vi "HGCalSensorTestingPanel3.vi"() -> ()   [LabVIEW 2015]
uses:
  <vilib>/Utility/file.llb/Read Delimited Spreadsheet (DBL).vi
  <vilib>/Utility/file.llb/Write Delimited Spreadsheet (string).vi
panel:
  out "XY Graph 3":cluster{"Y":dbl[], "Y":dbl[]}[](graph)
  out "HP count":u32
  in  "HP read count":u32
  in  "HP VISA":refnum<visa-resource-name>
  out "K237 count":u32
  in  "K237 VISA":refnum<visa-resource-name>
  out "XY Graph 2":cluster{"Y":dbl[], "Y":dbl[]}[](graph)
  out "return count 5":u32
  in  "write buffer 2":string
  out "return count 4":u32
  in  "QT VISA":refnum<visa-resource-name>
  in  "write buffer":string
  out "return count 3":u32
  in  "byte count 2":u32
  out "XY Graph":cluster{"Y":dbl[], "Y":dbl[]}[](graph)
  out "return count":u32
  in  "K706 VISA":refnum<visa-resource-name>
  in  "Measurement Data":string[][](table)
  in  "OK Button":bool
  in  "Delay (s):":dbl
  in  "Channel:":dbl
  in  "Voltage (V):":dbl
  out "Channel:":dbl format="%#3_6g"
  out "mV(nA)":dbl
  out "pF":dbl
  out "V":dbl
  out "nA":dbl
  # "C"
  # "A"
  # "V"
  # "1M"
  # "1M"
  # "Single Measurement"
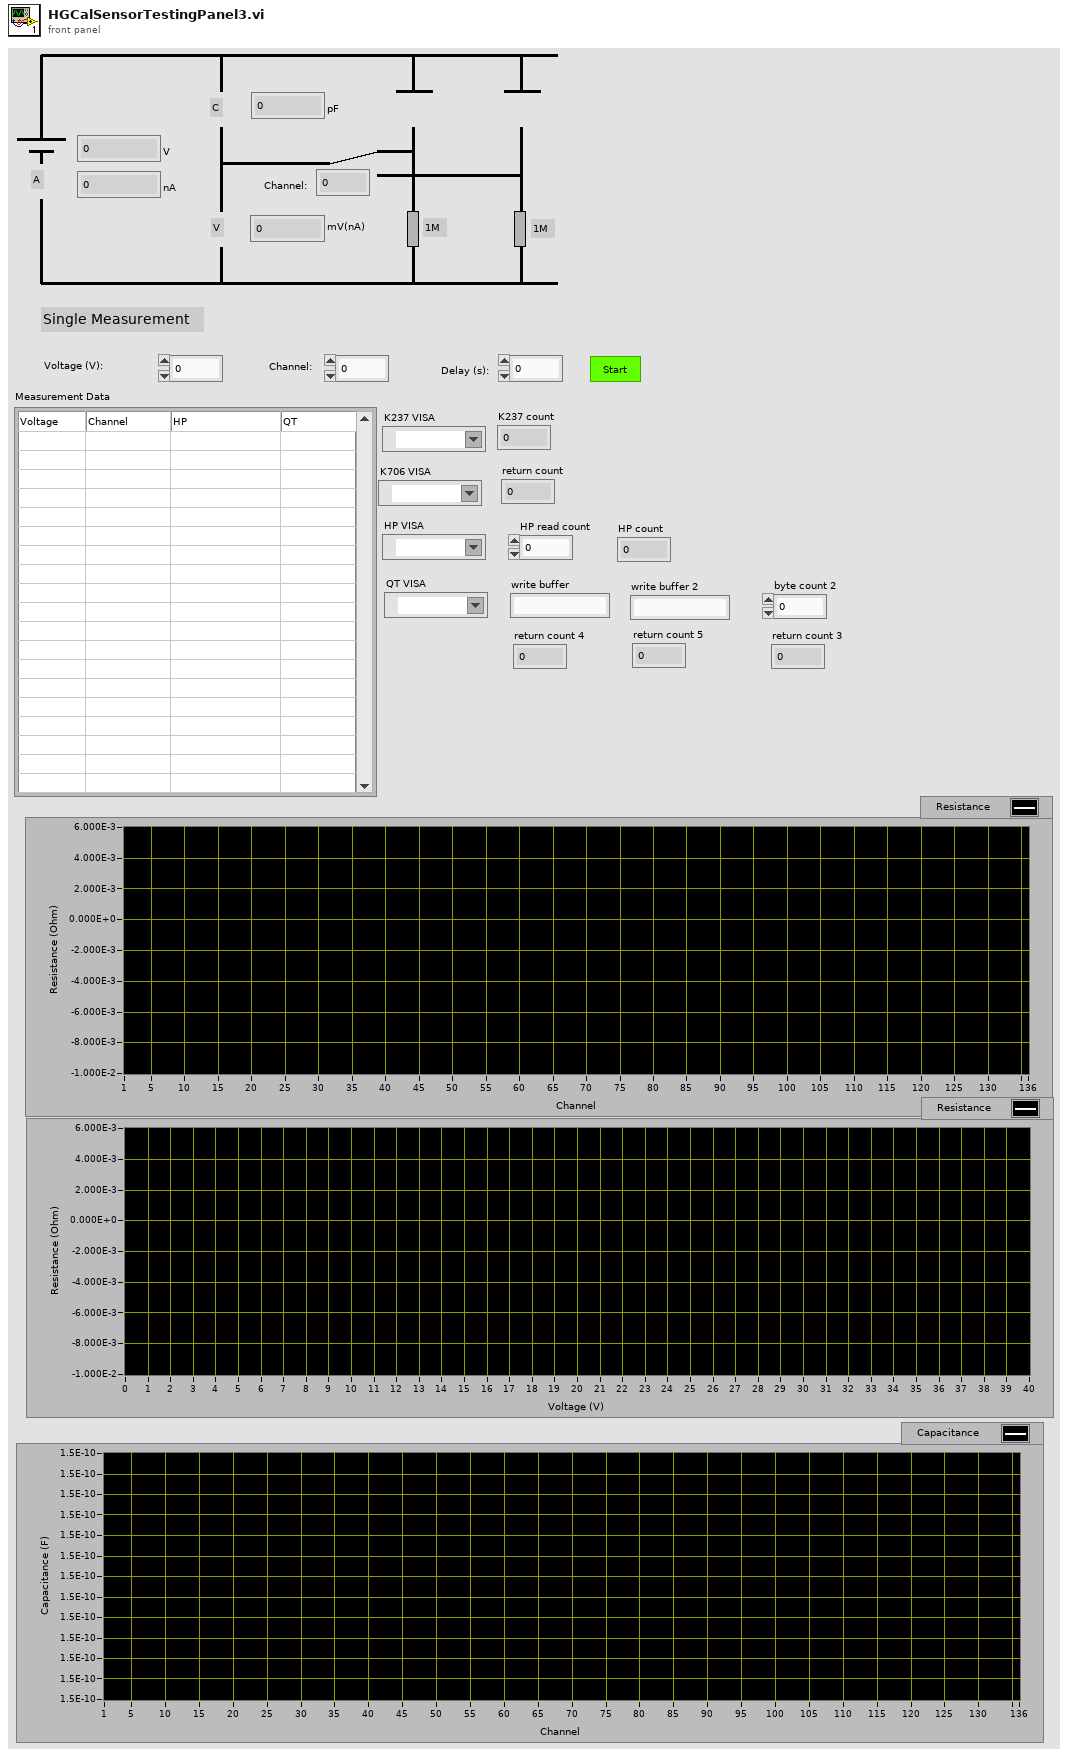
[diagram p1: front panel]
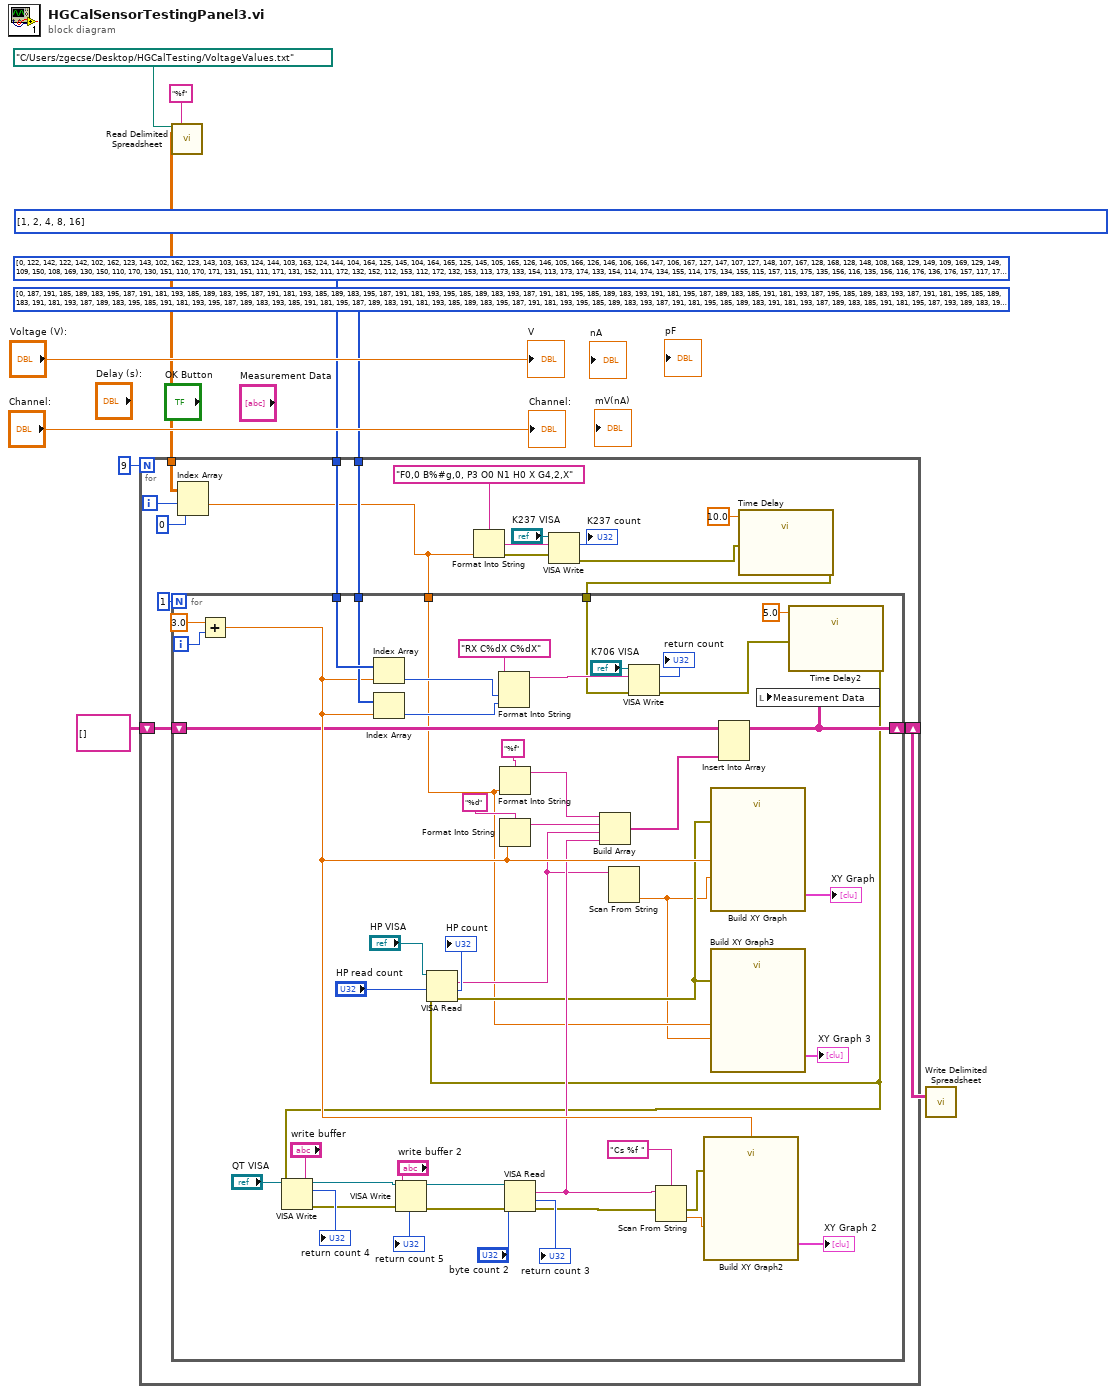
[diagram p0: block diagram]
diagram:
  (unwired) i32[] [1, 2, 4, 8, 16]
  n1 = call-poly <vilib>:"Read Delimited Spreadsheet.vi"("file path (dialog if empty)"=path "C:/Users/zgecse/Desktop/HGCalTesting/VoltageValues.txt", "format (%.3f)"="%f") -> ("all rows"=w1:dbl[][])  [unwired: 8 in, 5 out]
  n2 = for {
    N: 9 -> [_]
    tunnel: i32[] [0, 122, 142, 122, 142, 102, 162, 123, 143, 102, 162, 123, 143, 103, 163, 124, 144, 103, 163, 124, 144, 104, 164, 125, 145, 104, 164, 165, 125, 145, 105, 165, 126, 146, 105, 166, 126, 146, 106, 166, 147, 106, 167, 127, 147, 107, 127, 148, 107, 167, 128, 168, 128, 148, 108, 168, 129, 149, 109, 169, 129, 149, 109, 150, 108, 169, 130, 150, 110, 170, 130, 151, 110, 170, 171, 131, 151, 111, 171, 131, 152, 111, 172, 132, 152, 112, 153, 112, 172, 132, 153, 113, 173, 133, 154, 113, 173, 174, 133, 154, 114, 174, 134, 155, 114, 175, 134, 155, 115, 157, 115, 175, 135, 156, 116, 135, 156, 116, 176, 136, 176, 157, 117, 177, 136, 158, 117, 177, 137, 137, 158, 118, 178, 138, 138, 159, 178] -> [w24]
    tunnel: i32[] [0, 187, 191, 185, 189, 183, 195, 187, 191, 181, 193, 185, 189, 183, 195, 187, 191, 181, 193, 185, 189, 183, 195, 187, 191, 181, 193, 195, 185, 189, 183, 193, 187, 191, 181, 195, 185, 189, 183, 193, 191, 181, 195, 187, 189, 183, 185, 191, 181, 193, 187, 195, 185, 189, 183, 193, 187, 191, 181, 195, 185, 189, 183, 191, 181, 193, 187, 189, 183, 195, 185, 191, 181, 193, 195, 187, 189, 183, 193, 185, 191, 181, 195, 187, 189, 183, 191, 181, 193, 185, 189, 183, 195, 187, 191, 181, 193, 195, 185, 189, 183, 193, 187, 191, 181, 195, 185, 189, 183, 191, 181, 193, 187, 189, 183, 185, 191, 181, 195, 187, 193, 189, 183, 195, 185, 191, 181, 193, 187, 185, 189, 183, 195, 187, 185, 191, 193] -> [w23]
    shift-right: [w25] -> w7
    shift-left: string[][] [] -> [w27]
    tunnel: w1 -> [w15]
    i -> [w17]
    n3 = Index Array(array=w15, index (row)=w17, index (col)=0 ("disabled index (col)")) -> (element=w16:dbl)
    n4 = Format Into String(format string="F0,0 B%#g,0, P3 O0 N1 H0 X G4,2,X" ("F0,0X B%f,0,X L%f,0X P3X O0X"), w16) -> (resulting string=w18:string, error out=w19:errorcluster)  [unwired: 2 in]
    n5 = VISA Write(VISA resource name="K237 VISA", write buffer=w18, error in (no error)=w19) -> (return count=→"K237 count":u32, error out=w13:errorcluster)  [unwired: 1 out]
    n6 = call "Time Delay"("error in (no error)"=w13, "Delay Time (s)"=10.0) -> ("error out"=w12:errorcluster)  [unwired: 9 in]
    n7 = for {
      N: 1 -> [_]
      shift-right: [w39] -> w25
      shift-left: w27 -> [w40]
      tunnel: w24 -> [w69]
      tunnel: w23 -> [w68]
      tunnel: w12 -> [w41]
      tunnel: w16 -> [w30]
      i -> [w70]
      n8 = Add(x=3.0, y=w70) -> (x+y=w47:dbl)
      n9 = Index Array(array=w69, index=w47) -> (element=w67:i32)
      n10 = Index Array(array=w68, index=w47) -> (element=w66:i32)
      n11 = Format Into String(format string="RX C%dX C%dX", w67, w66) -> (resulting string=w63:string)  [unwired: 2 in, 1 out]
      n12 = Format Into String(format string="%f", w30) -> (resulting string=w75:string)  [unwired: 2 in, 1 out]
      n13 = Format Into String(format string="%d", w47) -> (resulting string=w61:string)  [unwired: 2 in, 1 out]
      n14 = VISA Write(VISA resource name="K706 VISA", write buffer=w63, error in (no error)=w41) -> (return count=→"return count":u32, error out=w37:errorcluster)  [unwired: 1 out]
      n15 = call "Time Delay2"("error in (no error)"=w37, "Delay Time (s)"=5.0) -> ("error out"=w32:errorcluster)  [unwired: 9 in]
      n16 = VISA Write(VISA resource name="QT VISA", write buffer="write buffer", error in (no error)=w32) -> (VISA resource name out=w50:refnum<visa-resource-name>, return count=→"return count 4":u32, error out=w52:errorcluster)
      n17 = VISA Write(VISA resource name=w50, write buffer="write buffer 2", error in (no error)=w52) -> (VISA resource name out=w49:refnum<visa-resource-name>, return count=→"return count 5":u32, error out=w51:errorcluster)
      n18 = VISA Read(VISA resource name="HP VISA", byte count="HP read count", error in (no error)=w32) -> (read buffer=w33:string, return count=→"HP count":u32, error out=w31:errorcluster)  [unwired: 1 out]
      n19 = VISA Read(VISA resource name=w49, byte count="byte count 2", error in (no error)=w51) -> (read buffer=w45:string, return count=→"return count 3":u32, error out=w44:errorcluster)  [unwired: 1 out]
      n20 = Build Array(w75, w61, w33, w45) -> (w74:string[])
      n21 = Scan From String(input string=w33) -> (output 1=w29:dbl)  [unwired: 4 in, 3 out]
      n22 = Scan From String(format string="Cs %f ", input string=w45, error in=w44) -> (error out=w43:errorcluster, output 1=w46:dbl)  [unwired: 2 in, 2 out]
      n23 = call "Build XY Graph2"("error in (no error)"=w43, "Y Input"=w46, "X Input"=w47) -> ("XY Graph"=→"XY Graph 2":cluster{"X":dbl[], "Y":dbl[]}[])  [unwired: 7 in, 1 out]
      n24 = call "Build XY Graph"("error in (no error)"=w31, "Y Input"=w29, "X Input"=w47) -> ("XY Graph"=→"XY Graph":cluster{"X":dbl[], "Y":dbl[]}[])  [unwired: 7 in, 1 out]
      n25 = call "Build XY Graph3"("error in (no error)"=w31, "Y Input"=w29, "X Input"=w30) -> ("XY Graph"=→"XY Graph 3":cluster{"X":dbl[], "Y":dbl[]}[])  [unwired: 7 in, 1 out]
      n26 = Insert Into Array(array=w40, new element=w74) -> (w39:string[][])  [unwired: 2 in]
      n27 = local write "Measurement Data"(w39) -> ()
    }
  }
  n28 = call-poly <vilib>:"Write Delimited Spreadsheet.vi"("2D data"=w7) -> ()  [unwired: 13 in, 2 out]
  "V" <- "Voltage (V):"
  "Channel:" <- "Channel:"
